vi "channeldata_2groups.vi"() -> ()   [LabVIEW 2019]
panel:
  out "Error Out":errorcluster
  in  "TDMS File":path=path "C:/Python/projects/nitdms/tests/tdms_files/channeldata_2groups.tdms"
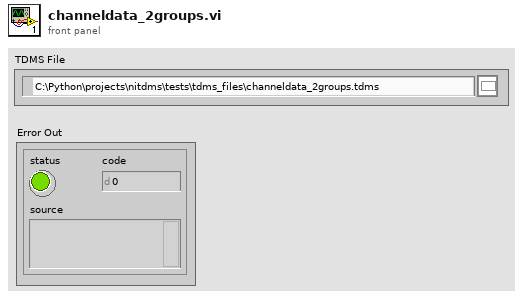
[diagram p1: front panel]
types:
  T1 = enum16{"open", "open or create", "create or replace", "create", "open (read-only)"}
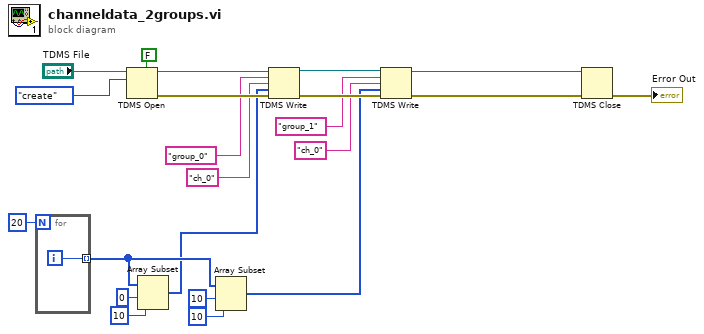
[diagram p0: block diagram]
diagram:
  n1 = for {
    N: 20 -> [_]
    tunnel: [w23] -> w11 mode=indexing
    i -> [w23]
  }
  n2 = TDMS Open(5:FALSE ("create index file? (T)"), 10:T1."create" ("operation (0:open)"), 11:"TDMS File") -> (0:w18:errorcluster, 3:w17:refnum<k34>)  [unwired: 4 in]
  n3 = Array Subset(array=w11, index=0, length=10) -> (w8:i32[])
  n4 = Array Subset(array=w11, index=10, length=10) -> (w1:i32[])
  n5 = TDMS Write(0:w17, 5:"group_0", 7:"ch_0", 9:w8, 11:w18) -> (4:w6:refnum<k34>, 15:w7:errorcluster)  [unwired: 1 in, 2 out]
  n6 = TDMS Write(0:w6, 5:"group_1", 7:"ch_0", 9:w1, 11:w7) -> (4:w4:refnum<k34>, 15:w5:errorcluster)  [unwired: 1 in, 2 out]
  n7 = TDMS Close(8:w5, 11:w4) -> (0:→"Error Out":errorcluster)  [unwired: 1 out]
